vi "Find Image by name.vi"(8 "error in (no error)":errorcluster, 10 "Imagename":string, 11 "EmbedImage in":refnum<class "EmbedImage.lvclass">) -> (0 "error out":errorcluster, 3 "EmbedImage out":refnum<class "EmbedImage.lvclass">)   [LabVIEW 2023, in "EmbedImage.lvlib" / "EmbedImage.lvclass"]
uses:
  Library/EmbedImage.lvclass
  Custom Controls/Image Types.ctl
  Library/EmbedImage.lvclass/EmbedImage.ctl
panel:
  out "dup path":path
  in  "Image Types":T1
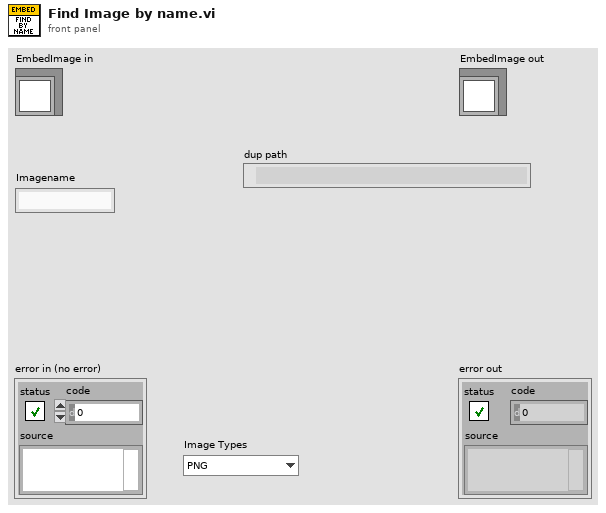
[diagram p1: front panel]
types:
  T1 = typedef "EmbedImage.lvlib/EmbedImage.lvclass/Image Types.ctl" = enum16{"PNG", "JPG", "JPEG", "BMP"}
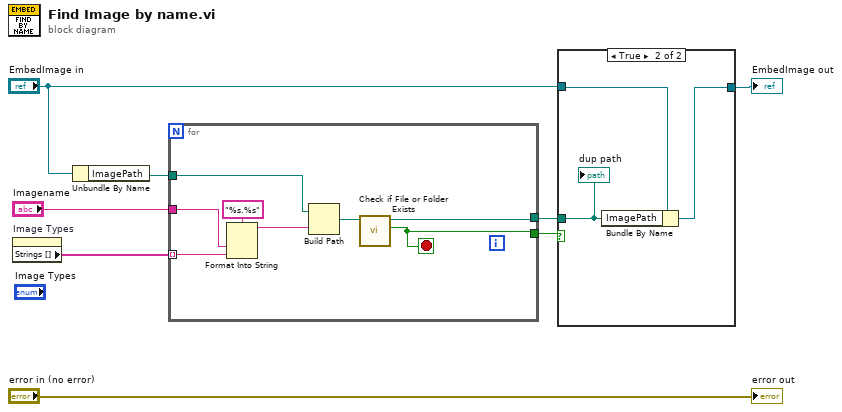
[diagram p0: block diagram]
diagram:
  n1 = property on="Image Types" class="Enum (strict)"() -> ("Strings []"=w8:string[])  [unwired: 2 in, 2 out]
  n2 = Unbundle By Name("EmbedImage in") -> ("ImagePath"=w1:path)
  n3 = for {
    tunnel: w8 -> [w14] mode=indexing
    tunnel: "Imagename" -> [w15]
    tunnel: w1 -> [w13]
    tunnel: [w10] -> w4
    tunnel: [w9] -> w3
    stop <- w9 stop-if-true
    n4 = Format Into String(format string="%s.%s", w15, w14) -> (resulting string=w12:string)  [unwired: 2 in, 1 out]
    n5 = Build Path(base path=w13, name or relative path=w12) -> (appended path=w11:path)
    n6 = call <vilib>:"Check if File or Folder Exists.vi"("path"=w11) -> ("file or folder exists?"=w9:bool, "dup path"=w10:path)  [unwired: 8 in, 1 out]
  }
  n7 = case shown="True" w3 {
    tunnel: "EmbedImage in" -> [w17 w20]
    tunnel: [w17 w19] -> w5
    tunnel: w4 -> [_ w18]
    frame False {
    }
    frame True {
      n8 = Bundle By Name(cluster=w20, "ImagePath"=w18) -> (w19:refnum<class "EmbedImage.lvclass">)
      "dup path" <- w18
    }
  }
  "EmbedImage out" <- w5
  "error out" <- "error in (no error)"
